vi "Global 1.vi"() -> ()   [LabVIEW 2016]
panel:
  out "state":fxp<+/-,25,16>
  out "Time":u32
  out "Count(uSec)":fxp<+/-,25,16>
  out "stop":bool
  in  "SampleRight":i16
  out "n":i64
  out "Address":i64
  out "Gain Comb 1":fxp<+/-,25,16>
  in  "SampleLeft":i16
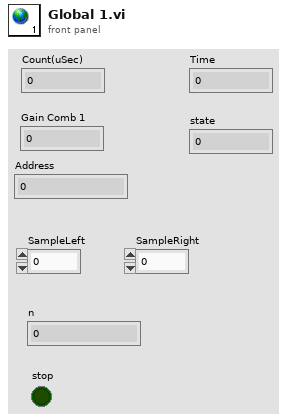
[diagram p1: front panel]
diagram:
